vi "Actor Core.vi"(8 "error in":errorcluster, 11 "Application Manager in":refnum<class "Application Manager.lvclass">) -> (0 "error out":errorcluster, 3 "Actor out":refnum<class "Actor.lvclass">)   [LabVIEW 2020, in "Application Manager.lvlib" / "Application Manager.lvclass"]
doc: "<p>(<strong>Filename</strong>: <span class=\"dnl\">Actor Framework.lvlib:Actor.lvclass:Actor Core.vi</span>)</p>\n<p>Receives messages to the actor, reacts to them, and initiates any error handling that may shut the actor down.</p>\n<p>Descendant classes may override this VI to append parallel tasks for the actor to complete while it handles messages. Overrides use the <a href=\"nihelplauncher://docs/csh?context=lvcore_glang_udclass\">Call Parent Class Method</a> node.</p>"
uses:
  Application Manager.lvclass
  C:/Program Files/National Instruments/LabVIEW 2026/vi.lib/ActorFramework/Actor/Actor.lvclass
  <vilib>/ActorFramework/Actor/Actor.lvclass
  TDMS Data Source/TDMS Data Source/TDMS Data Source.lvclass
  Simple UI/Simple UI/Simple UI.lvclass
  CPU FFT Calculator/CPU FFT Calculator/CPU FFT Calculator.lvclass
  GPU FFT Calculator/GPU FFT Calculator/GPU FFT Calculator.lvclass
  <vilib>/Natan Biesmans/G2CPU GPU and CPU HPC Toolkit/ArrayFire Driver/TypeDefs/backend.ctl
  Simple UI/Simple UI/GPU Batch Results.ctl
  CPU FFT Calculator/CPU FFT Calculator/CPU Metrics.ctl
  Application Manager.lvclass/Application Manager.ctl
  GPU FFT Calculator/GPU FFT Calculator Messages/Set GPU Msg/Set GPU Msg.lvclass/Set GPU Msg.ctl
  <vilib>/ActorFramework/Message Enqueuer/Message Enqueuer.lvclass/Message Enqueuer.ctl
  <vilib>/ActorFramework/Message Enqueuer/Enqueue.vi
  GPU FFT Calculator/GPU FFT Calculator Messages/Set GPU Msg/Set GPU Msg.lvclass
  C:/Program Files/National Instruments/LabVIEW 2026/vi.lib/ActorFramework/Message/Message.lvclass
  <vilib>/ActorFramework/Message Priority Queue/Priority Enqueue.vi
  Generic Actor/Generic Actor/Generic Actor.lvclass
  <vilib>/Natan Biesmans/G2CPU GPU and CPU HPC Toolkit/ArrayFire Driver/AF.lvlib
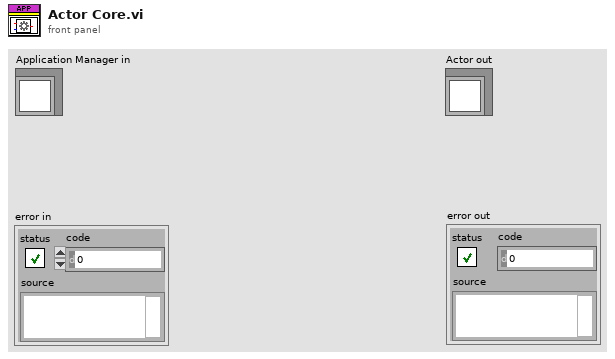
[diagram p1: front panel]
types:
  T1 = typedef "Simple UI.lvlib/Simple UI.lvclass/CPU Metrics.ctl" = cluster{"FFT Time":dbl, "Throughput":dbl, "Queue Depth":u64, "Elapsed Time":dbl}
  T2 = typedef "Simple UI.lvlib/Simple UI.lvclass/GPU Batch Results.ctl" = cluster{"Queue Depth":dbl, "Throughput":dbl, "Upload Speed":dbl, "Elapsed Time":dbl, "Throughput Valid":bool}
  T3 = typedef "AF.lvlib/backend.ctl" = u32
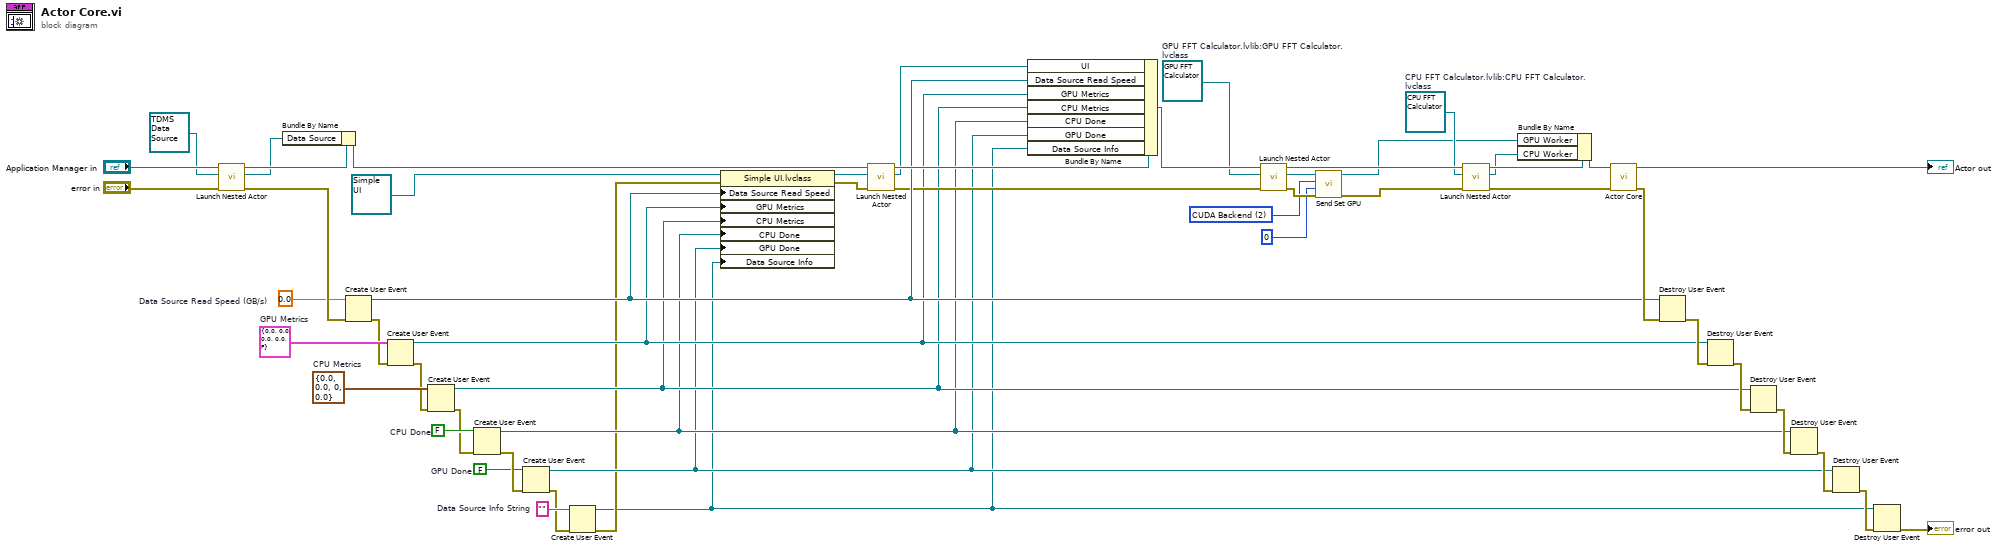
[diagram p0: block diagram]
diagram:
  w6 = ""  # Data Source Info String
  w11 = FALSE  # GPU Done
  w14 = FALSE  # CPU Done
  w18 = T1 {"FFT Time"=0.0, "Throughput"=0.0, "Queue Depth"=0, "Elapsed Time"=0.0}  # CPU Metrics
  w22 = T2 {"Queue Depth"=0.0, "Throughput"=0.0, "Upload Speed"=0.0, "Elapsed Time"=0.0, "Throughput Valid"=FALSE}  # GPU Metrics
  w24 = T3 2 items=["Default Backend"=0, "CPU Backend"=1, "CUDA Backend"=2, "OPENCL Backend"=4, "Intel OneAPI Backend"=8] ("Backend")
  w30 = refnum<class "GPU FFT Calculator.lvclass"> refnum  # GPU FFT Calculator.lvlib:GPU FFT Calculator.lvclass
  w29 = refnum<class "CPU FFT Calculator.lvclass"> refnum  # CPU FFT Calculator.lvlib:CPU FFT Calculator.lvclass
  w44 = 0.0  # Data Source Read Speed (GB/s)
  n1 = call <vilib>:"Launch Nested Actor.vi"("error in (no error)"="error in", "Nested Actor"=refnum<class "TDMS Data Source.lvclass"> refnum ("TDMS Data Source.lvlib:TDMS Data Source.lvclass"), "Caller Actor in"="Application Manager in") -> ("error out"=w45:errorcluster, "Nested Actor's Enqueuer"=w38:refnum<class "Message Enqueuer.lvclass">, "Caller Actor out"=w49:refnum<class "Application Manager.lvclass">)  [unwired: 6 in]
  n2 = Bundle By Name(cluster=w49, "Data Source"=w38) -> (w39:refnum<class "Application Manager.lvclass">)
  n3 = Create User Event(user event datatype=w44, error in=w45) -> (user event=w40:refnum<user-event>, error out=w21:errorcluster)
  n4 = Create User Event(user event datatype=w22, error in=w21) -> (user event=w19:refnum<user-event>, error out=w17:errorcluster)
  n5 = Create User Event(user event datatype=w18, error in=w17) -> (user event=w15:refnum<user-event>, error out=w13:errorcluster)
  n6 = Create User Event(user event datatype=w14, error in=w13) -> (user event=w8:refnum<user-event>, error out=w12:errorcluster)
  n7 = Create User Event(user event datatype=w11, error in=w12) -> (user event=w7:refnum<user-event>, error out=w5:errorcluster)
  n8 = Create User Event(user event datatype=w6, error in=w5) -> (user event=w1:refnum<user-event>, error out=w4:errorcluster)
  n9 = property class="Simple UI.lvclass"(reference=refnum<class "Simple UI.lvclass"> refnum ("Simple UI.lvlib:Simple UI.lvclass"), error in=w4, "Data Source Read Speed"=w40, "GPU Metrics"=w19, "CPU Metrics"=w15, "CPU Done"=w8, "GPU Done"=w7, "Data Source Info"=w1) -> (reference out=w42:refnum<class "Simple UI.lvclass">, error out=w41:errorcluster)
  n10 = call <vilib>:"Launch Nested Actor.vi"("error in (no error)"=w41, "Nested Actor"=w42, "Caller Actor in"=w39) -> ("error out"=w37:errorcluster, "Nested Actor's Enqueuer"=w46:refnum<class "Message Enqueuer.lvclass">, "Caller Actor out"=w48:refnum<class "Application Manager.lvclass">)  [unwired: 6 in]
  n11 = Bundle By Name(cluster=w48, "UI"=w46, "Data Source Read Speed"=w40, "GPU Metrics"=w19, "CPU Metrics"=w15, "CPU Done"=w8, "GPU Done"=w7, "Data Source Info"=w1) -> (w36:refnum<class "Application Manager.lvclass">)
  n12 = call <vilib>:"Launch Nested Actor.vi"("error in (no error)"=w37, "Nested Actor"=w30, "Caller Actor in"=w36) -> ("error out"=w26:errorcluster, "Nested Actor's Enqueuer"=w28:refnum<class "Message Enqueuer.lvclass">, "Caller Actor out"=w34:refnum<class "Application Manager.lvclass">)  [unwired: 6 in]
  n13 = call "Send Set GPU.vi"("error in (no error)"=w26, "Device ID"=0, "Backend"=w24, "Message Enqueuer"=w28) -> ("error out"=w25:errorcluster, "Message Enqueuer out"=w27:refnum<class "Message Enqueuer.lvclass">)  [unwired: 6 in]
  n14 = call <vilib>:"Launch Nested Actor.vi"("error in (no error)"=w25, "Nested Actor"=w29, "Caller Actor in"=w34) -> ("error out"=w33:errorcluster, "Nested Actor's Enqueuer"=w31:refnum<class "Message Enqueuer.lvclass">, "Caller Actor out"=w32:refnum<class "Application Manager.lvclass">)  [unwired: 6 in]
  n15 = Bundle By Name(cluster=w32, "GPU Worker"=w27, "CPU Worker"=w31) -> (w35:refnum<class "Application Manager.lvclass">)
  n16 = call-parent "Actor Core.vi"("error in"=w33, "Actor in"=w35) -> ("error out"=w43:errorcluster, "Actor out"=→"Actor out":refnum<class "Actor.lvclass">)  [unwired: 8 in]
  n17 = Destroy User Event(user event=w40, error in=w43) -> (error out=w20:errorcluster)
  n18 = Destroy User Event(user event=w19, error in=w20) -> (error out=w16:errorcluster)
  n19 = Destroy User Event(user event=w15, error in=w16) -> (error out=w10:errorcluster)
  n20 = Destroy User Event(user event=w8, error in=w10) -> (error out=w9:errorcluster)
  n21 = Destroy User Event(user event=w7, error in=w9) -> (error out=w3:errorcluster)
  n22 = Destroy User Event(user event=w1, error in=w3) -> (error out=→"error out":errorcluster)
